vi "GetClockSettings.vi"(0 "object in":refnum<class "Experiment2.lvclass">, 5 "error in (no error)":errorcluster) -> (14 "object out":refnum<class "Experiment2.lvclass">, 16 "DOClockSettings":T3, 19 "error out":errorcluster)   [LabVIEW 2024, in "Experiment2.lvclass"]
uses:
  Experiment2.lvclass
  AD2_DO_SDK_class/DOTrigger.ctl
  AD2_WFG_SDK_class/AD2TriggerSources.ctl
  Experiment2.lvclass/Experiment2.ctl
  AD2_SDK_class/AD2_SDK.lvclass
  AD2_DO_SDK_class/AD2_DO_SDK.lvclass
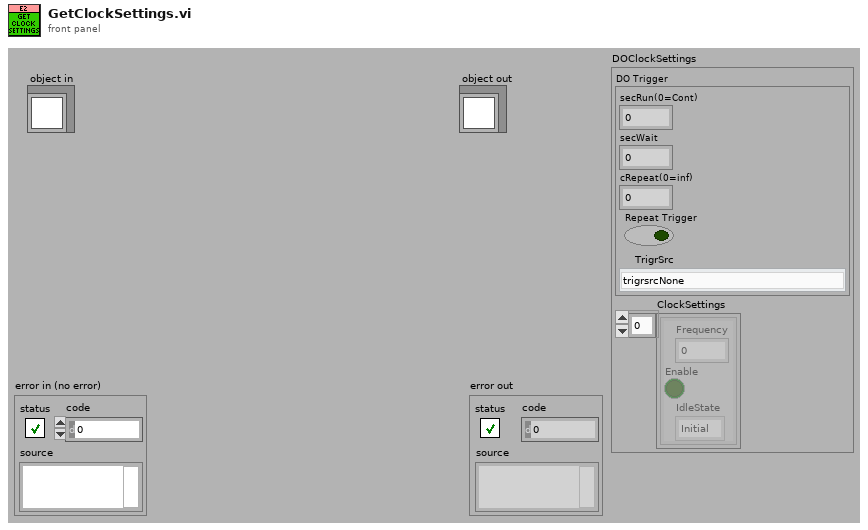
[diagram p1: front panel]
types:
  T1 = typedef "AD2_DO_SDK.lvclass/DOTrigger.ctl" = cluster{"secRun(0=Cont)":dbl, "secWait":dbl, "cRepeat(0=inf)":i32, "Repeat Trigger":bool, "TrigrSrc":T2}
  T2 = typedef "AD2_SDK.lvclass/AD2TriggerSources.ctl" = enum8{"trigrsrcNone", "trigsrcPC", "trigsrcDetectorAnalogIn", "trigsrcDetectorDigitalIn", "trigsrcAnalogIn", "trigsrcDigitalIn", "trigsrcDigitalOut", "trigsrcAnalogOut1", "trigsrcAnalogOut2", "trigsrcAnalogOut3", "trigsrcAnalogOut4", "trigsrcExternal1", "trigsrcExternal2", "trigsrcExternal3", "trigsrcExternal4", ""}
  T3 = cluster{"DO Trigger":T1, "ClockSettings":cluster{"Frequency":dbl, "Enable":bool, "IdleState":enum16{"Initial", "Low", "High", "Z"}}[]}
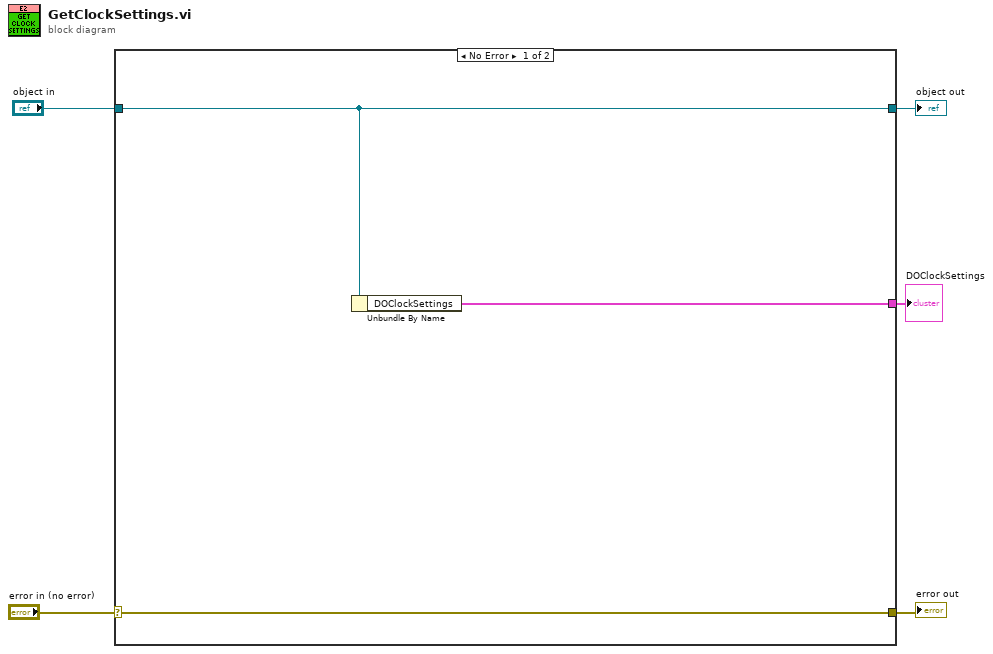
[diagram p0: block diagram]
diagram:
  n1 = case shown="No Error" "error in (no error)" {
    selector: "error in (no error)" -> [w7 w10]
    tunnel: [w7 w10] -> w4
    tunnel: [w6 w9] -> w2
    tunnel: "object in" -> [w6 w9]
    tunnel: [w8 _] -> w1
    frame No Error {
      n2 = Unbundle By Name(w6) -> ("DOClockSettings"=w8:T3)
    }
    frame Error {
    }
  }
  "error out" <- w4
  "object out" <- w2
  "DOClockSettings" <- w1
